vi "set status tags.vi"(5 "ns since last call":u64, 6 "late count in":u32, 7 "desired dt ns":u64, 8 "status reporting":T1={"late index (bool)"=-1, "late count (U32)"=-1, "current dt ns(U64)"=-1, "synchronous modules"=[], "asynchronous modules"=[]}, 9 "async module info in":T13, 10 "Module Info In":T3, 11 "Engine Tags In":T5) -> (1 "async module info out":T13, 2 "Module Info Out":T3, 3 "Engine Tags Out":T5, 4 "late count out":u32)   [LabVIEW 2013, in "Standard Engine Runtime.lvclass"]
doc: "This VI writes to any of the timing or error tags that have been configured based on the results of this iteration of the loop."
uses:
  Standard Engine Runtime.lvclass
  <vilib>/NI/Tag Bus/table/data table.ctl
  async execution info.ctl
  asynchronous process data.ctl
  async command notification.ctl
  <vilib>/NI/Tag Bus Module Framework/runtime/execution settings.ctl
  async error info.ctl
  <vilib>/NI/Tag Bus Module Framework/runtime/error classification.ctl
  Data Table with Transfer Spec.ctl
  <vilib>/NI/Tag Bus/table/transfer specification.ctl
  <vilib>/NI/Tag Bus/tag/Data Type.ctl
  Configuration/Module Decimation.ctl
  Configuration/Module Error Configuration.ctl
  Configuration/Error Actions By Category.ctl
  Configuration/Error Actions.ctl
  Module Execution Info.ctl
  <vilib>/NI/Tag Bus Module Framework/runtime/TBM module execution interface.lvclass
  status reporting data.ctl
  module status reporting.ctl
  <vilib>/NI/Tag Bus/table/data polymorphs/write one/write Boolean.vi
  <vilib>/NI/Tag Bus/table/data polymorphs/write one/write U32.vi
  <vilib>/NI/Tag Bus/table/data polymorphs/write one/write U64.vi
  <vilib>/NI/Tag Bus/table/data polymorphs/write one/write I32.vi
  <vilib>/NI/Tag Bus/table/data table.lvlib
  <vilib>/NI/Tag Bus/tag/tag descriptor.lvclass
  Configuration/Standard Engine Configuration.lvclass
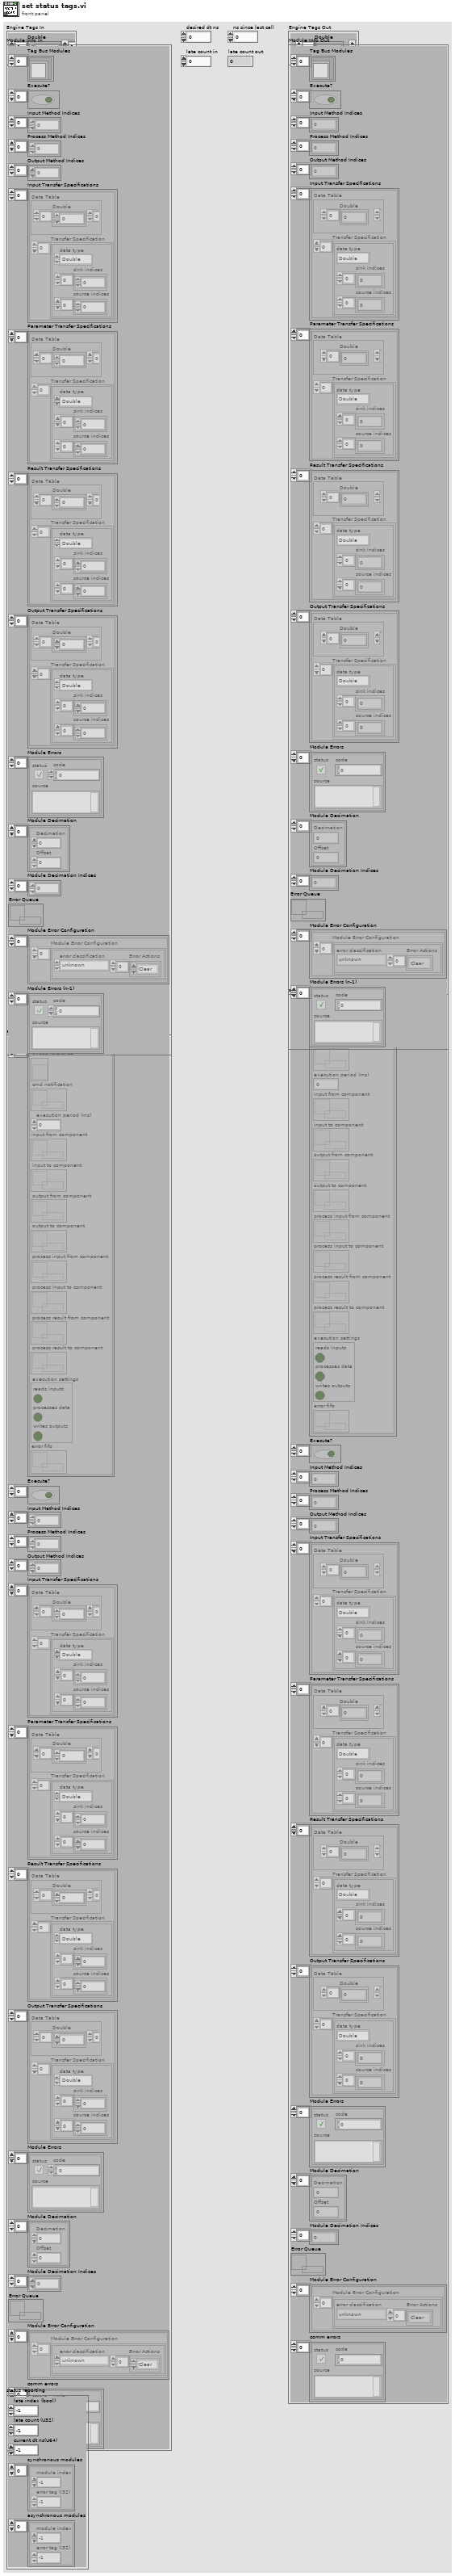
[diagram p1: front panel]
types:
  T1 = typedef "Standard Engine Runtime.lvclass/status reporting data.ctl" = cluster{"late index (bool)":i32, "late count (U32)":i32, "current dt ns(U64)":i32, "synchronous modules":T2[], "asynchronous modules":T2[]}
  T2 = typedef "Standard Engine Runtime.lvclass/module status reporting.ctl" = cluster{"module index":i32, "error tag (I32)":i32}
  T3 = typedef "Standard Engine Runtime.lvclass/Module Execution Info.ctl" = cluster{"Tag Bus Modules":refnum<class "TBM module execution interface.lvclass">[], "Execute?":bool[], "Input Method Indices":i32[], "Process Method Indices":i32[], "Output Method Indices":i32[], "Input Transfer Specifications":T4[], "Parameter Transfer Specifications":T4[], "Result Transfer Specifications":T4[], "Output Transfer Specifications":T4[], "Module Errors":errorcluster[], "Module Decimation":T8[], "Module Decimation Indices":i32[], "Error Queue":refnum<queue>, "Module Error Configuration":T9[], "Module Errors (n-1)":errorcluster[]}
  T4 = typedef "Standard Engine Runtime.lvclass/Data Table with Transfer Spec.ctl" = cluster{"Data Table":T5, "Transfer Specification":T6[]}
  T5 = typedef "tag bus.lvlib/data table.lvlib/data table.ctl" = cluster{"Double":dbl[], "Single":sgl[], "I64":i64[], "I32":i32[], "I16":i16[], "I8":i8[], "U64":u64[], "U32":u32[], "U16":u16[], "U8":u8[], "Boolean":bool[], "String":string[], "Array of Double":cluster{"DBL Array":dbl[]}[], "Array of Single":cluster{"SGL Array":sgl[]}[], "Array of I64":cluster{"I64 Array":i64[]}[], "Array of I32":cluster{"I32 Array":i32[]}[], "Array of I16":cluster{"I16 Array":i16[]}[], "Array of I8":cluster{"I8 Array":i8[]}[], "Array of U64":cluster{"U64 Array":u64[]}[], "Array of U32":cluster{"U32 Array":u32[]}[], "Array of U16":cluster{"U16 Array":u16[]}[], "Array of U8":cluster{"U8 Array":u8[]}[], "Array of Boolean":cluster{"Boolean Array":bool[]}[], "Array of String":cluster{"String Array":string[]}[]}
  T6 = typedef "tag bus.lvlib/data table.lvlib/transfer specification.ctl" = cluster{"data type":T7, "sink indices":i32[], "source indices":i32[]}
  T7 = typedef "tag bus.lvlib/tag descriptor.lvclass/Data Type.ctl" = enum16{"Double", "Single", "I64", "I32", "I16", "I8", "U64", "U32", "U16", "U8", "Boolean", "String", "Array of Double", "Array of Single", "Array of I64", "Array of I32", "Array of I16", "Array of I8", "Array of U64", "Array of U32", "Array of U16", "Array of U8", "Array of Boolean", "Array of String"}
  T8 = typedef "Standard Engine Configuration.lvclass/Module Decimation.ctl" = cluster{"Decimation":u16, "Offset":u16}
  T9 = typedef "Standard Engine Configuration.lvclass/Module Error Configuration.ctl" = cluster{"Module Error Configuration":T10[]}
  T10 = typedef "Standard Engine Configuration.lvclass/Error Actions By Category.ctl" = cluster{"error classification":T11, "Error Actions":T12[]}
  T11 = typedef "TBM module execution interface.lvclass/error classification.ctl" = enum16{"unknown", "none", "trivial", "recoverable", "critical"}
  T12 = typedef "Standard Engine Configuration.lvclass/Error Actions.ctl" = enum16{"Clear", "Notify", "Stop Component", "Stop Engine", "Safe State", "Attempt Recovery"}
  T13 = typedef "Standard Engine Runtime.lvclass/async execution info.ctl" = cluster{"Tag Bus Modules":T14[], "Execute?":bool[], "Input Method Indices":i32[], "Process Method Indices":i32[], "Output Method Indices":i32[], "Input Transfer Specifications":T4[], "Parameter Transfer Specifications":T4[], "Result Transfer Specifications":T4[], "Output Transfer Specifications":T4[], "Module Errors":errorcluster[], "Module Decimation":T8[], "Module Decimation Indices":i32[], "Error Queue":refnum<queue>, "Module Error Configuration":T9[], "comm errors":errorcluster[]}
  T14 = typedef "Standard Engine Runtime.lvclass/asynchronous process data.ctl" = cluster{"thread reference":refnum<vi>, "cmd notification":refnum<k33>, "execution period (ms)":i32, "input from component":refnum<queue>, "input to component":refnum<queue>, "output from component":refnum<queue>, "output to component":refnum<queue>, "process input from component":refnum<queue>, "process input to component":refnum<queue>, "process result from component":refnum<queue>, "process result to component":refnum<queue>, "execution settings":T15, "error fifo":refnum<k33>}
  T15 = typedef "TBM module execution interface.lvclass/execution settings.ctl" = cluster{"reads inputs":bool, "processes data":bool, "writes outputs":bool}
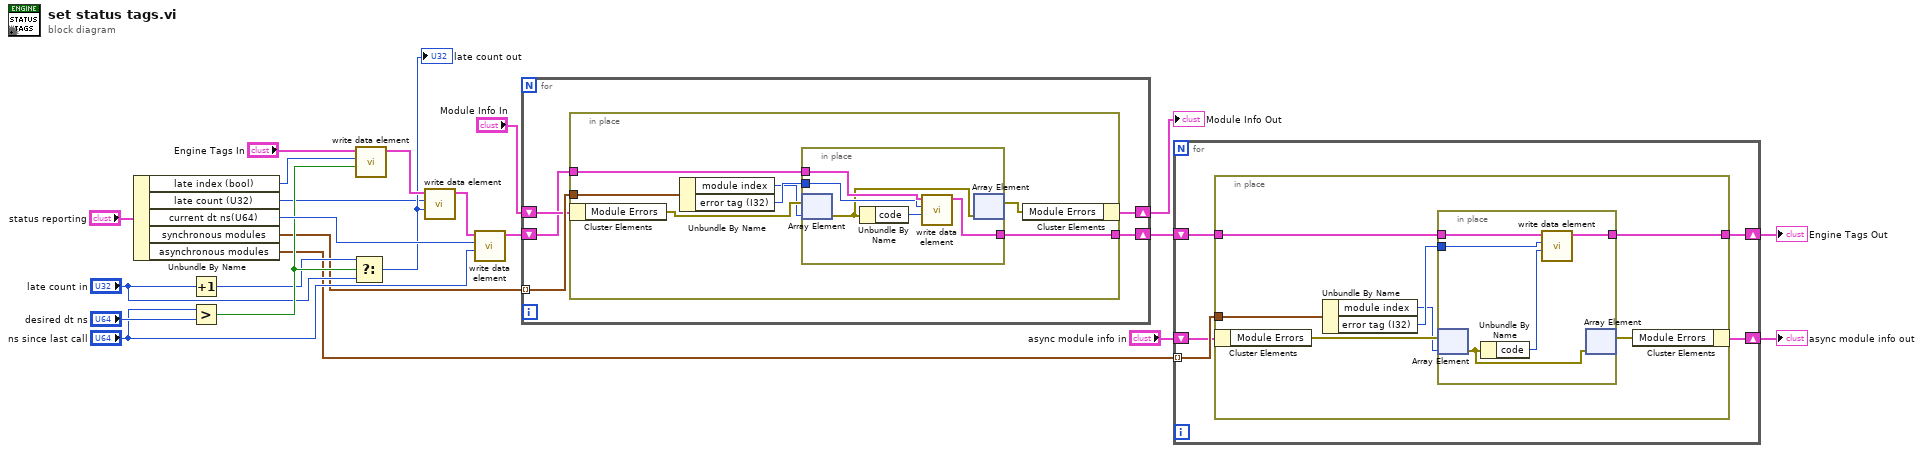
[diagram p0: block diagram]
diagram:
  n1 = Unbundle By Name("status reporting") -> ("late index (bool)"=w18:i32, "late count (U32)"=w10:i32, "current dt ns(U64)"=w16:i32, "synchronous modules"=w7:T2[], "asynchronous modules"=w3:T2[])
  n2 = Increment(x="late count in") -> (x+1=w13:u32)
  n3 = Greater?(x="ns since last call", y="desired dt ns") -> (0:w14:bool)
  n4 = Select(t=w13, s=w14, f="late count in") -> (s? t:f=w11:u32)
  "late count out" <- w11
  n5 = call-poly <vilib>:"write data element.vi"("value"=w14, "index"=w18, "data table in"="Engine Tags In") -> ("data table out"=w20:T5)  [unwired: 8 in]
  n6 = call-poly <vilib>:"write data element.vi"("value"=w11, "index"=w10, "data table in"=w20) -> ("data table out"=w17:T5)  [unwired: 8 in]
  n7 = call-poly <vilib>:"write data element.vi"("value"="ns since last call", "index"=w16, "data table in"=w17) -> ("data table out"=w6:T5)  [unwired: 8 in]
  n8 = for {
    shift-right: [w25] -> w9
    shift-left: "Module Info In" -> [w26]
    tunnel: w7 -> [w27] mode=indexing
    shift-right: [w23] -> w1
    shift-left: w6 -> [w24]
    n9 = in-place {
      in-place-border: w27 -> [w34]
      in-place-border: w24 -> [w31]
      in-place-border: [w30] -> w23
      n10 = in-place-cluster #1(w26) -> ("Module Errors"=w32:errorcluster[])
      n11 = Unbundle By Name(w34) -> ("module index"=w28:i32, "error tag (I32)"=w29:i32)
      n12 = in-place {
        in-place-border: w31 -> [w39]
        in-place-border: [w38] -> w30
        in-place-border: w29 -> [w37]
        n13 = in-place-array #2(w32, w28) -> (w36:errorcluster)
        n14 = Unbundle By Name(w36) -> ("code"=w35:i32)
        n15 = call-poly <vilib>:"write data element.vi"("value"=w35, "index"=w37, "data table in"=w39) -> ("data table out"=w38:T5)  [unwired: 8 in]
        n16 = in-place-array #2(w36) -> (w33:errorcluster[])  [unwired: 1 out]
      }
      n17 = in-place-cluster #1("Module Errors"=w33) -> (w25:T3)
    }
  }
  "Module Info Out" <- w9
  n18 = for {
    shift-right: [w42] -> w5
    shift-left: "async module info in" -> [w43]
    tunnel: w3 -> [w44] mode=indexing
    shift-right: [w40] -> w2
    shift-left: w1 -> [w41]
    n19 = in-place {
      in-place-border: w44 -> [w51]
      in-place-border: w41 -> [w48]
      in-place-border: [w47] -> w40
      n20 = in-place-cluster #3(w43) -> ("Module Errors"=w49:errorcluster[])
      n21 = Unbundle By Name(w51) -> ("module index"=w45:i32, "error tag (I32)"=w46:i32)
      n22 = in-place {
        in-place-border: w48 -> [w56]
        in-place-border: [w55] -> w47
        in-place-border: w46 -> [w54]
        n23 = in-place-array #4(w49, w45) -> (w53:errorcluster)
        n24 = Unbundle By Name(w53) -> ("code"=w52:i32)
        n25 = call-poly <vilib>:"write data element.vi"("value"=w52, "index"=w54, "data table in"=w56) -> ("data table out"=w55:T5)  [unwired: 8 in]
        n26 = in-place-array #4(w53) -> (w50:errorcluster[])  [unwired: 1 out]
      }
      n27 = in-place-cluster #3("Module Errors"=w50) -> (w42:T13)
    }
  }
  "Engine Tags Out" <- w2
  "async module info out" <- w5
